vi "Initialization VI.vi"(8 "error in (no error)":errorcluster, 10 "Custom XML":string, 11 "Device Item Ref in":T1 format="%.0x") -> (0 "error out":errorcluster, 3 "Device Item Ref out":T1 format="%.0x")   [LabVIEW 2015, in "Engine Simulation Toolkit System Explorer.lvlib"]
uses:
  Engine Simulation Toolkit System Explorer.lvlib
  <vilib>/NI Veristand/Custom Device API/Custom Device Item Ref.ctl
  <vilib>/NI Veristand/Custom Device API/Custom Device Channel Type.ctl
  <vilib>/NI Veristand/Custom Device API/Custom Device Loop Type.ctl
  <vilib>/NI Veristand/Custom Device API/Custom Device Timed Loop Priority.ctl
  Shared/Constants and GUIDs.vi
  <vilib>/NI Veristand/Custom Device API/Custom Device API.lvlib
  Shared/Engine Simulation Toolkit Shared.lvlib
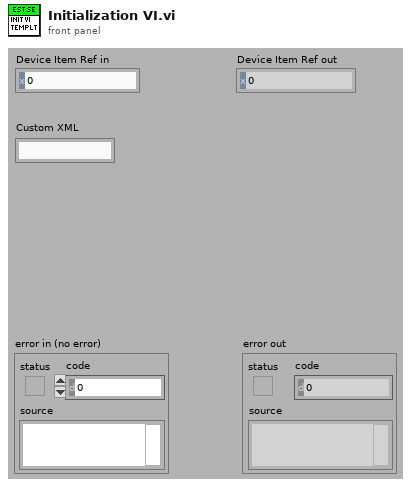
[diagram p1: front panel]
types:
  T1 = typedef "Custom Device API.lvlib/Custom Device Item Ref.ctl" = u64
  T2 = typedef "Custom Device API.lvlib/Custom Device Timed Loop Priority.ctl" = enum32{"Low", "Medium", "High"}
  T3 = typedef "Custom Device API.lvlib/Custom Device Loop Type.ctl" = enum32{"While Loop", "Timed Loop"}
  T4 = typedef "Custom Device API.lvlib/Custom Device Channel Type.ctl" = enum16{"Input", "Output"}
  T5 = typedef "Engine Simulation Toolkit Shared.lvlib/Channel.ctl" = cluster{"Name":string, "Units":string, "Default":dbl, "Description":string}
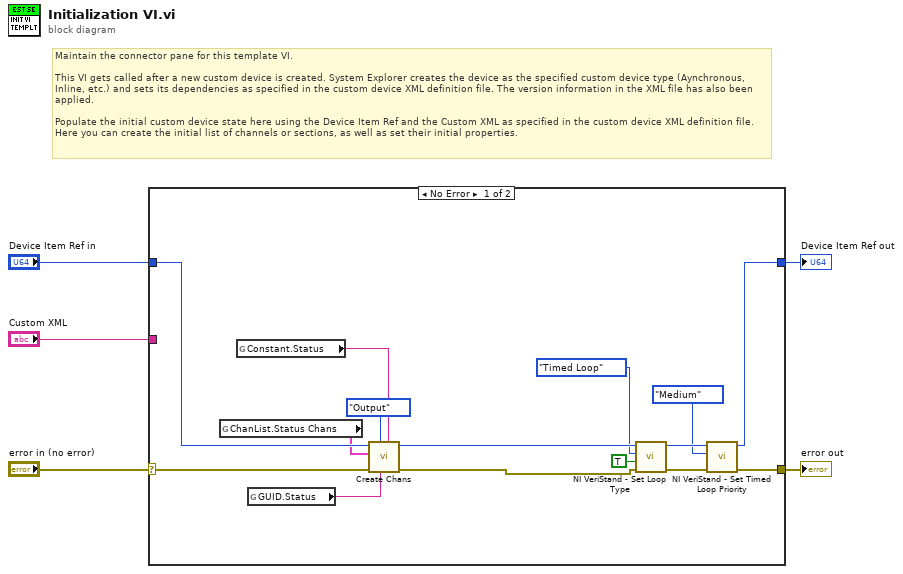
[diagram p0: block diagram]
diagram:
  # "Maintain the connector pane for this template VI.\n\nThis VI gets called after a new custom device is created. System Explorer creates the device as the specified custom device type (Aynchronous, Inline, etc.) and sets its dependencies as specified in the custom device XML definition file. The version information in the XML file has also been applied.\n\nPopulate the initial custom device state here using the Device Item Ref and the Custom XML as specified in the custom device XML definition file. Here you can create the initial list of channels or sections, as well as set their initial properties."
  n1 = case shown="No Error" "error in (no error)" {
    selector: "error in (no error)" -> [w20 w22]
    tunnel: [w11 w22] -> w5
    tunnel: [w9 w21] -> w3
    tunnel: "Device Item Ref in" -> [w18 w21]
    tunnel: "Custom XML" -> [_ _]
    frame No Error {
      n2 = global read "Constants and GUIDs.vi" "ChanList.Status Chans"() -> (w16:T5[])
      n3 = global read "Constants and GUIDs.vi" "Constant.Status"() -> (w7:string)
      n4 = global read "Constants and GUIDs.vi" "GUID.Status"() -> (w6:string)
      n5 = call "Create Chans.vi"("New Section Name (none)"=w7, "new section GUID (\"\":del prot)"=w6, "Type"=Custom_Device_Channel_Type."Output", "error in (no error)"=w20, "Channels"=w16, "Section Ptr"=w18) -> ("error out"=w19:errorcluster, "Section Ptr dup"=w15:T1)  [unwired: 2 in, 2 out]
      n6 = call <vilib>:"NI VeriStand - Set Loop Type.vi"("error in (no error)"=w19, "Use Device Clock (Timed Loops only)"=TRUE, "Loop type"=Custom_Device_Loop_Type."Timed Loop", "Device Ref in"=w15) -> ("error out"=w14:errorcluster, "Device Ref out"=w10:T1)  [unwired: 6 in]
      n7 = call <vilib>:"NI VeriStand - Set Timed Loop Priority.vi"("error in (no error)"=w14, "Priority"=Custom_Device_Timed_Loop_Priority."Medium", "Device Ref in"=w10) -> ("error out"=w11:errorcluster, "Device Ref out"=w9:T1)  [unwired: 7 in]
    }
    frame Error {
    }
  }
  "error out" <- w5
  "Device Item Ref out" <- w3
